vi "FPGA Init.vi"   [LabVIEW 2014]
uses:
  <vilib>/rvi/DataTransferAndStorage/Container/XNode/niFpgaContainer.xnode
  <vilib>/Utility/file.llb/Read From Spreadsheet File (I64).vi
  <vilib>/rvi/interface/nirviOpenFPGA/nirviOpenFPGA.xnode
  <vilib>/rvi/interface/nirviMethod/nirviMethod.xnode
  <vilib>/FPGAPlugInAG/Dynamic/niLvFpga_Run_Dynamic.vi
  <vilib>/rvi/Memory/Memory_Emulation/nirvimemoryFastEmulation.vi
  <vilib>/rvi/Memory/Memory_Emulation/nirvimemoryEmulation.vi
  Wave generator.vi
  <vilib>/rvi/interface/RandomDataEmulation/nirviRandomDataOpen.vi
  <vilib>/rvi/interface/common/niFpgaCacheSessionInfoDynamic.vi
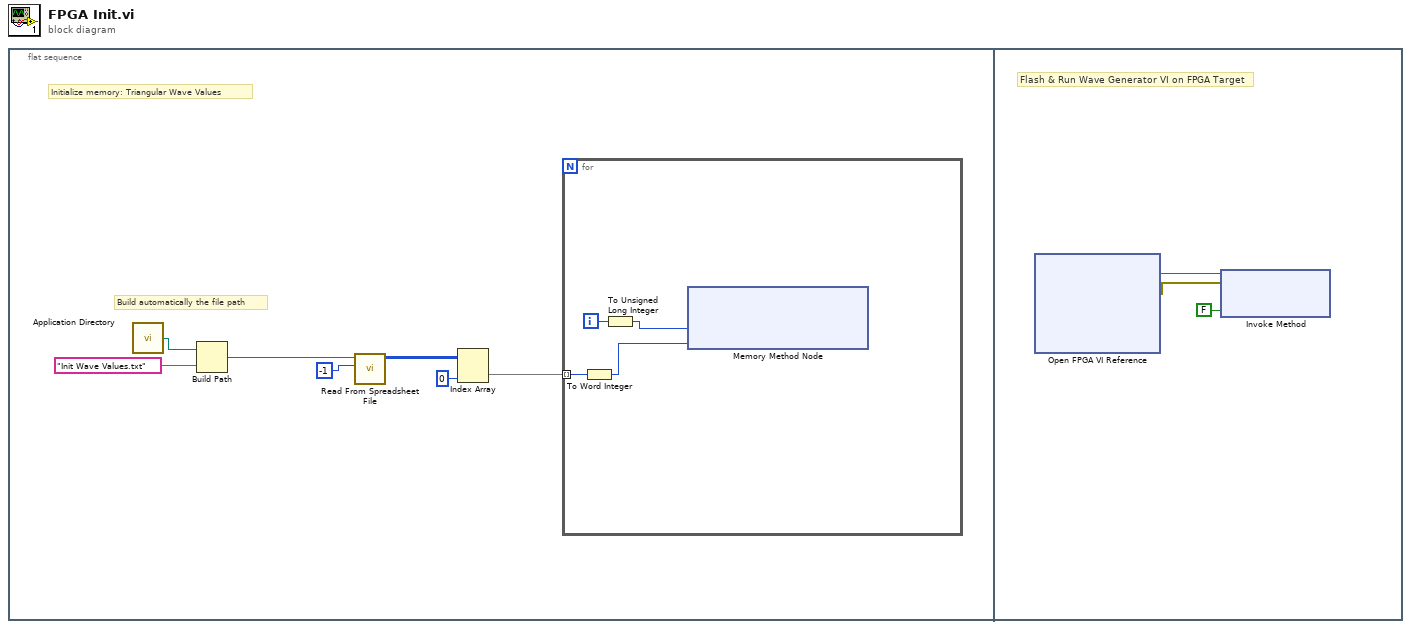
[diagram p0: block diagram]
diagram:
  n1 = flat-sequence {
    frame #0 {
      # "Initialize memory: Triangular Wave Values"
      # "Build automatically the file path"
      n2 = call <vilib>:"Application Directory.vi"() -> ("Application Directory"=w3:path)
      n3 = Build Path(base path=w3, name or relative path="Init Wave Values.txt") -> (appended path=w1:path)
      n4 = call-poly <vilib>:"Read From Spreadsheet File.vi"("number of rows (all:-1)"=-1, "file path (dialog if empty)"=w1) -> ("all rows"=w6:i64[][])  [unwired: 5 in, 4 out]
      n5 = Index Array(array=w6, index (col)=0 ("disabled index (col)")) -> (element=w4:i64[])  [unwired: 1 in]
      n6 = for {
        tunnel: w4 -> [w11] mode=indexing
        i -> [w9]
        n7 = To Word Integer(number=w11) -> (16bit integer=w10:i16)
        n8 = To Unsigned Long Integer(number=w9) -> (unsigned 32bit integer=w8:u32)
        n9 = xnode ("Memory Method Node")("Address"=w8, "Data"=w10) -> ()  [unwired: 1 in, 1 out]
      }
    }
    frame #1 {
      # "Flash & Run Wave Generator VI on FPGA Target"
      n10 = xnode "Open FPGA VI Reference"() -> ("FPGA VI Reference Out"=w14:refnum<k20>, "error out"=w13:errorcluster)  [unwired: 2 in]
      n11 = xnode "Invoke Method"("FPGA VI Reference In"=w14, "error in"=w13, "Wait Until Done (F)"=FALSE) -> ()  [unwired: 2 out]
    }
  }
